vi "Create (DB).vi"(4 "Polygon Threshold (Default 0.5)":sgl=0.5, 5 "Unclip Ratio (Default: 2.0)":dbl=2.0, 6 "Binary Threshold (Default 0.3)":sgl=0.3, 7 "Max Candidates (Default: 50)":u16=50, 8 "error in (no error)":errorcluster, 11 "Model":T1) -> (0 "error out":errorcluster, 3 "Text Detector":refnum<class "Text Detector.lvclass">)   [LabVIEW 2020, in "feature_detection.lvlib" / "Text Detector.lvclass"]
doc: "Create a DNN based DB type Text Detector. See for more details https://docs.opencv.org/4.11.0/db/d0f/classcv_1_1dnn_1_1TextDetectionModel__DB.html"
uses:
  Text Detector.lvclass
  Model.ctl
  common/Image Size (Integer).ctl
  common/Object Point (Float).ctl
  Text Detector.lvclass/Text Detector.ctl
  Path to String Path.vi
  common/common.lvlib
  common/bin/gartoolkit_dnn_32-1.dll
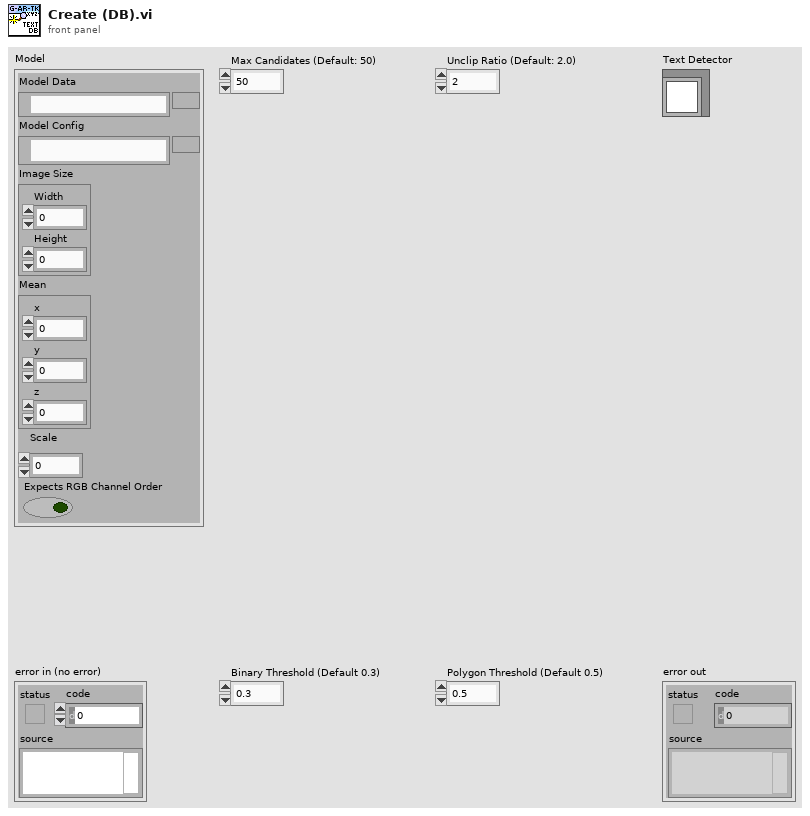
[diagram p1: front panel]
types:
  T1 = typedef "feature_detection.lvlib/Text Detector.lvclass/Model.ctl" = cluster{"Model Data":path, "Model Config":path, "Image Size":T2, "Mean":T3, "Scale":dbl, "Expects RGB Channel Order":bool}
  T2 = typedef "common.lvlib/Image Size (Integer).ctl" = cluster{"Width":u16, "Height":u16}
  T3 = typedef "common.lvlib/Object Point (Float).ctl" = cluster{"x":dbl, "y":dbl, "z":dbl}
  T4 = cluster{"Model Data":string, "Model Config":string, "Image Size":T2, "Mean":T3, "Scale":dbl, "Expects RGB Channel Order":bool}
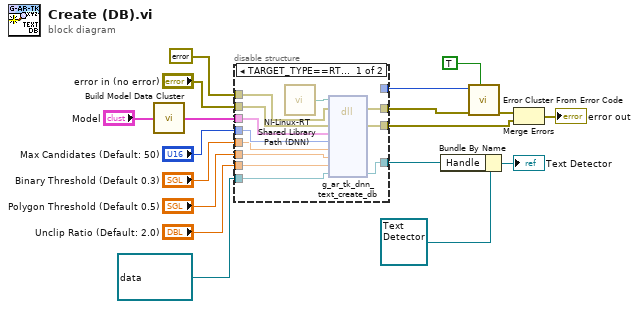
[diagram p0: block diagram]
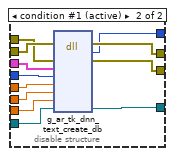
[diagram p2: hidden frame]
diagram:
  n1 = call "Build Model Data Cluster.vi"("Model in"="Model") -> ("Model out"=w1:T4)
  n2 = disable-structure "Conditional Disable Structure" shown="TARGET_TYPE==RT&&OS==Linux" {
    disable-tunnel: "error in (no error)" -> [w27 w42]
    disable-tunnel: errorcluster {"status"=FALSE, "code"=0, "source"=""} ("error constant") -> [w26 w41]
    disable-tunnel: refnum<data-value> refnum ("EDVR") -> [w20 w40]
    disable-tunnel: [w29 w39] -> w15
    disable-tunnel: [_ w38] -> w14
    disable-tunnel: [w19 w37] -> w13
    disable-tunnel: [w28 w36] -> w12
    disable-tunnel: "Unclip Ratio (Default: 2.0)" -> [w21 w35]
    disable-tunnel: "Polygon Threshold (Default 0.5)" -> [w22 w34]
    disable-tunnel: "Binary Threshold (Default 0.3)" -> [w23 w33]
    disable-tunnel: "Max Candidates (Default: 50)" -> [w24 w32]
    disable-tunnel: w1 -> [w25 w31]
    frame condition #0 {
      n3 = call "NI-Linux-RT Shared Library Path (DNN).vi"() -> ("Path"=w30:path)
      n4 = dll-call lib="?" fn="g_ar_tk_dnn_text_create_db" ("g_ar_toolkit.*.*:g_ar_tk_capture_context_create")(path in=w30, error in=w26, "error_cluster"=w27, "model"=w25, "max_candidates"=w24, "binary_threshold"=w23, "poly_threshold"=w22, "unclip_ratio"=w21, "EDVR"=w20) -> (error out=w29:errorcluster, "error_cluster"=w28:errorcluster, "EDVR"=w19:refnum<data-value>)  [unwired: 7 in, 1 out]
    }
    frame condition #1 (active) {
      n5 = dll-call lib="C:/serenial/lib/g-augmented-reality-toolkit/LabVIEW/common/bin/gartoolkit_dnn_*-1.*" fn="g_ar_tk_dnn_text_create_db" ("g_ar_toolkit.*.*:g_ar_tk_capture_context_create")(error in=w42, "error_cluster"=w41, "model"=w31, "max_candidates"=w32, "binary_threshold"=w33, "poly_threshold"=w34, "unclip_ratio"=w35, "EDVR"=w40) -> (error out=w39:errorcluster, w38:i32, "error_cluster"=w36:errorcluster, "EDVR"=w37:refnum<data-value>)  [unwired: 7 in, 1 out]
    }
  }
  n6 = Bundle By Name(cluster=refnum<class "Text Detector.lvclass"> refnum ("Text Detector in"), "Handle"=w13) -> (→"Text Detector":refnum<class "Text Detector.lvclass">)
  n7 = call <vilib>:"Error Cluster From Error Code.vi"("show call chain? (False)"=TRUE, "error in (no error)"=w15, "error code (0)"=w14) -> ("error out"=w18:errorcluster)  [unwired: 6 in]
  n8 = Merge Errors(w18, w12) -> (→"error out":errorcluster)
